vi "DataReader.vi"   [LabVIEW 2012]
uses:
  LVJumpEvent.ctl
  Globals.vi
types:
  T1 = typedef "LVJumpEvent.ctl" = cluster{"onTrampoline":bool, "timestamp":timestamp, "timestampMs":dbl}
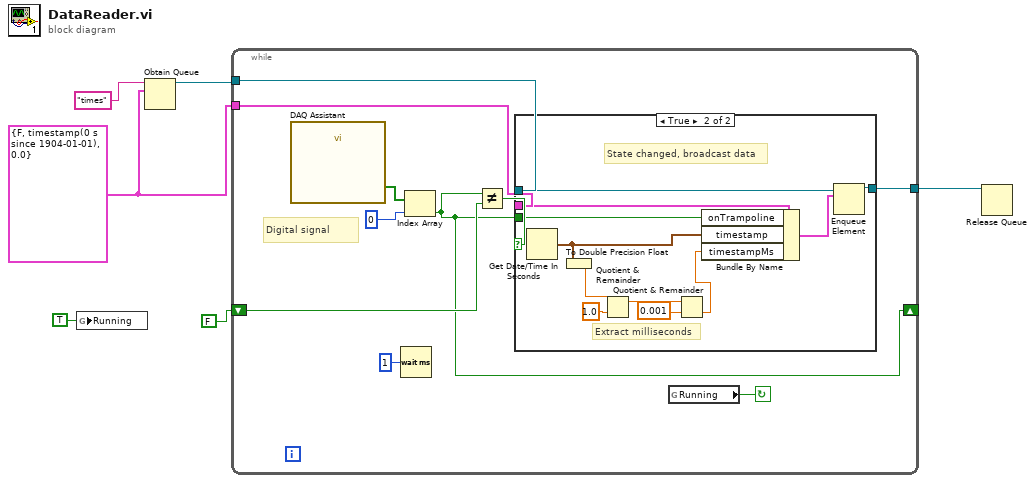
[diagram p0: block diagram]
diagram:
  w3 = T1 {"onTrampoline"=FALSE, "timestamp"=timestamp(0 s since 1904-01-01), "timestampMs"=0.0}
  n1 = global write "Globals.vi" "Running"(TRUE ("Running")) -> ()
  n2 = Obtain Queue(name (unnamed)="times", element data type=w3) -> (queue out=w4:refnum<queue>)  [unwired: 3 in, 2 out]
  n3 = while {
    shift-right: [w7] -> _
    shift-left: FALSE -> [w8]
    tunnel: w4 -> [w13]
    tunnel: w3 -> [w12]
    tunnel: [w9] -> w2
    stop <- w11 continue-if-true
    # "Digital signal"
    n4 = call "DAQ Assistant"() -> ("data"=w14:bool[])  [unwired: 17 in, 2 out]
    n5 = Wait (ms)(milliseconds to wait=u32 1) -> ()  [unwired: 1 out]
    n6 = Index Array(array=w14, index=0) -> (element=w7:bool)
    n7 = Not Equal?(x=w7, y=w8) -> (x != y?=w16:bool)
    n8 = case shown="True" w16 {
      tunnel: w13 -> [w17 w28]
      tunnel: w12 -> [_ w26]
      tunnel: w7 -> [_ w25]
      tunnel: [w17 w24] -> w9
      frame False {
      }
      frame True {
        # "Extract milliseconds"
        # "State changed, broadcast data"
        n9 = Get Date/Time In Seconds() -> (seconds since 1Jan1904=w19:timestamp)
        n10 = To Double Precision Float(number=w19) -> (double precision float=w22:dbl)
        n11 = Quotient & Remainder(x=w22, y=1.0) -> (x-y*floor(x/y)=w20:dbl)  [unwired: 1 out]
        n12 = Quotient & Remainder(x=w20, y=0.001) -> (floor(x/y)=w18:dbl)  [unwired: 1 out]
        n13 = Bundle By Name(cluster=w26, "onTrampoline"=w25, "timestamp"=w19, "timestampMs"=w18) -> (w27:T1)
        n14 = Enqueue Element(queue=w28, element=w27) -> (queue out=w24:refnum<queue>)  [unwired: 2 in, 2 out]
      }
    }
    n15 = global read "Globals.vi" "Running"() -> (w11:bool)
  }
  n16 = Release Queue(queue=w2) -> ()  [unwired: 2 in, 3 out]
